vi "Single_Measurement_Main_v1.vi"(7 "Config files paths":T1={"ZI config file (.ini)"="Config_Ver_1\\Zurich_params.ini", "Keithley config file (.ini)"="Config_Ver_1\\Keithley_params.ini", "Arduino config file (.ini)"="Config_Ver_1\\pulse_sequence.ini"}, 8 "error in":errorcluster, 10 "Timeout [ms]":u64=5000, 11 "Resources In":T2 {"ZI ModHandle"."ModHandle" format="0x%08x"; "ZI ModHandle"."Conn" format="0x%08x"; "ZI Handle"."Handle" format="0x%08x"; "ZI Handle"."Conn" format="0x%08x"}) -> (0 "error out":errorcluster, 3 "Resources Out":T2 {"ZI ModHandle"."ModHandle" format="0x%08x"; "ZI ModHandle"."Conn" format="0x%08x"; "ZI Handle"."Handle" format="0x%08x"; "ZI Handle"."Conn" format="0x%08x"})   [LabVIEW 2021]
uses:
  Resources.ctl
  <instrlib>/Zurich Instruments LabOne/Public/ziTypeHandle.ctl
  <instrlib>/Zurich Instruments LabOne/Public/Modules/ziTypeModHandle.ctl
  Config_File_Paths.ctl
  <instrlib>/Keithley 622x LV 2009/Typedefs/KE622x -- On Off Control.ctl
  <vilib>/Utility/error.llb/Error Cluster From Error Code.vi
  <vilib>/ErrorRing/Error Ring.xnode
  <instrlib>/Zurich Instruments LabOne/Zurich Instruments LabOne.lvlib
  <instrlib>/Keithley 622x LV 2009/Keithley 622x.lvlib
panel:
  out "progress":dbl(slide) scale=0.0..1.0
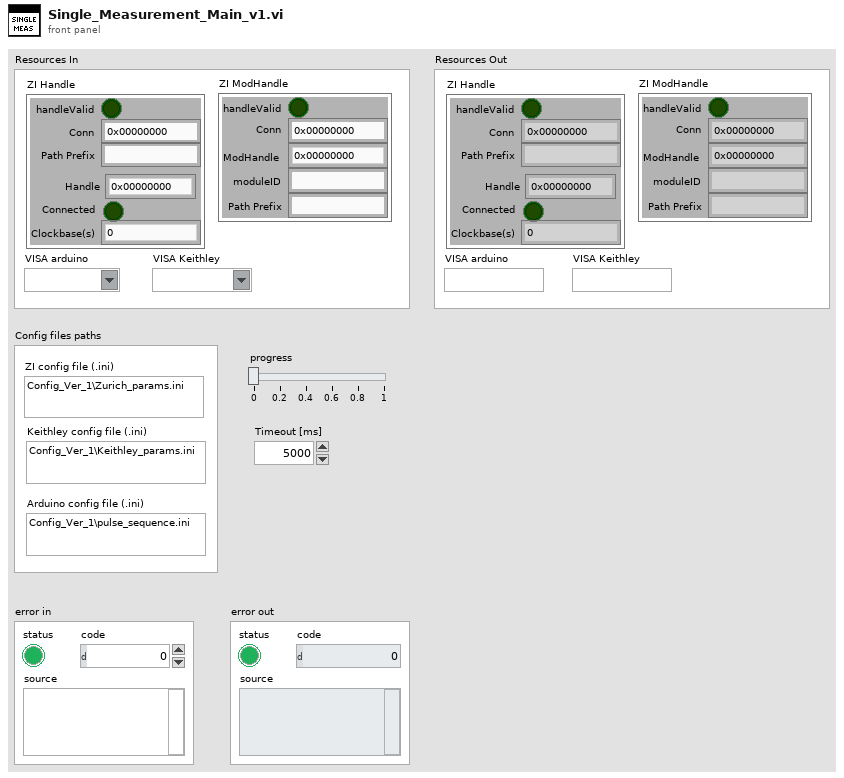
[diagram p1: front panel]
types:
  T1 = typedef "Config_File_Paths.ctl" = cluster{"ZI config file (.ini)":string, "Keithley config file (.ini)":string, "Arduino config file (.ini)":string}
  T2 = typedef "Resources.ctl" = cluster{"ZI Handle":T3, "ZI ModHandle":T4, "VISA arduino":refnum<visa-resource-name>, "VISA Keithley":refnum<visa-resource-name>}
  T3 = typedef "Zurich Instruments LabOne.lvlib/ziTypeHandle.ctl" = cluster{"handleValid":bool, "Conn":u64, "Path Prefix":string, "Handle":u64, "Connected":bool, "Clockbase(s)":dbl}
  T4 = typedef "Zurich Instruments LabOne.lvlib/ziTypeModHandle.ctl" = cluster{"handleValid":bool, "Conn":u64, "ModHandle":u64, "moduleID":string, "Path Prefix":string}
  T5 = typedef "Keithley 622x.lvlib/KE622x -- On Off Control.ctl" = enum16{"Off", "On"}
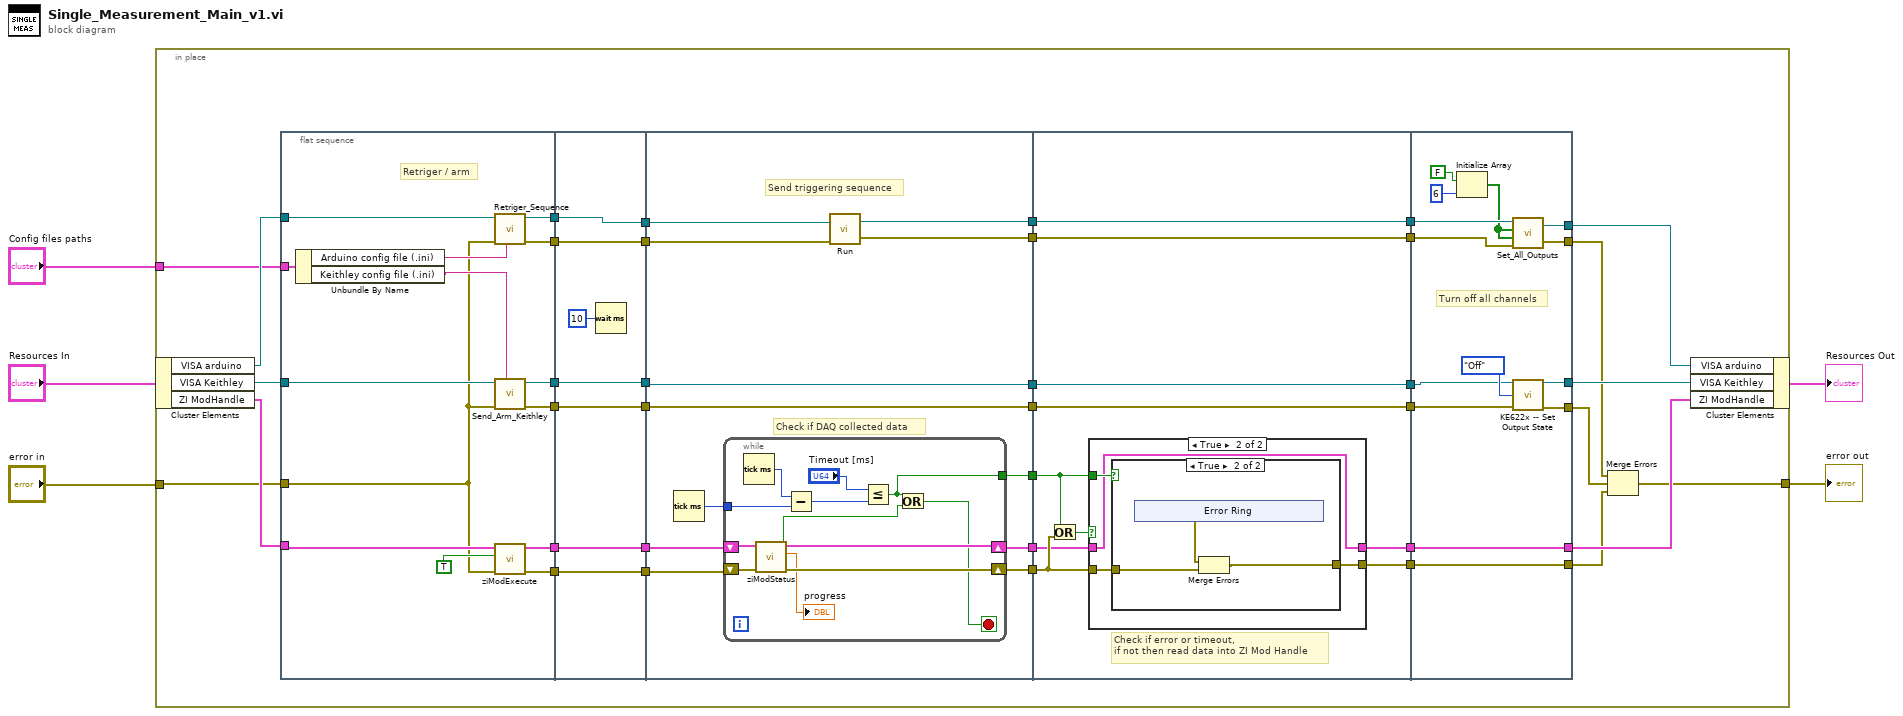
[diagram p0: block diagram]
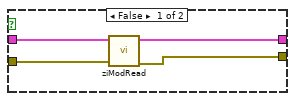
[diagram p2: hidden frame]
diagram:
  n1 = in-place {
    in-place-border: "Config files paths" -> [w39]
    in-place-border: "error in" -> [w38]
    in-place-border: [w6] -> w2
    n2 = in-place-cluster #1("Resources In") -> ("VISA arduino"=w40:refnum<visa-resource-name>, "VISA Keithley"=w41:refnum<visa-resource-name>, "ZI ModHandle"=w42:T4)
    n3 = flat-sequence {
      tunnel: w42 -> [w54]
      tunnel: w41 -> [w55]
      tunnel: w40 -> [w56]
      tunnel: w39 -> [w52]
      tunnel: w38 -> [w49]
      tunnel: [w48] -> w36
      tunnel: [w47] -> w34
      tunnel: [w46] -> w32
      tunnel: [w45] -> w30
      tunnel: [w44] -> w28
      tunnel: [w43] -> w26
      tunnel: [w62] -> w37
      tunnel: w36 -> [w62]
      tunnel: [w61] -> w35
      tunnel: w34 -> [w61]
      tunnel: [w60] -> w33
      tunnel: w32 -> [w60]
      tunnel: [w59] -> w31
      tunnel: w30 -> [w59]
      tunnel: [w58] -> w29
      tunnel: w28 -> [w58]
      tunnel: [w57] -> w27
      tunnel: w26 -> [w57]
      tunnel: w37 -> [w75]
      tunnel: w35 -> [w74]
      tunnel: w33 -> [w68]
      tunnel: w31 -> [w67]
      tunnel: w29 -> [w73]
      tunnel: w27 -> [w72]
      tunnel: [w70] -> w25
      tunnel: [w69] -> w24
      tunnel: [w68] -> w23
      tunnel: [w67] -> w22
      tunnel: [w66] -> w21
      tunnel: [w65] -> w20
      tunnel: [w64] -> w19
      tunnel: w25 -> [w97]
      tunnel: w24 -> [w96]
      tunnel: w23 -> [w95]
      tunnel: w22 -> [w94]
      tunnel: w21 -> [w91]
      tunnel: w20 -> [w90]
      tunnel: w19 -> [w92]
      tunnel: [w97] -> w18
      tunnel: [w96] -> w17
      tunnel: [w95] -> w16
      tunnel: [w94] -> w15
      tunnel: [w89] -> w14
      tunnel: [w88] -> w13
      tunnel: [w127] -> w9
      tunnel: [w128] -> w10
      tunnel: w18 -> [w121]
      tunnel: w17 -> [w119]
      tunnel: w16 -> [w125]
      tunnel: w15 -> [w124]
      tunnel: w14 -> [w128]
      tunnel: w13 -> [w127]
      tunnel: [w118] -> w11
      tunnel: [w117] -> w12
      tunnel: [w116] -> w7
      tunnel: [w115] -> w8
      frame #0 {
        # "Retriger / arm"
        n4 = Unbundle By Name(w52) -> ("Arduino config file (.ini)"=w51:string, "Keithley config file (.ini)"=w50:string)
        n5 = call "Retriger_Sequence.vi"("Filename (.ini)"=w51, "error in"=w49, "VISA arduino in"=w56) -> ("error out"=w48:errorcluster, "VISA arduino out"=w47:refnum<visa-resource-name>)  [unwired: 4 in, 3 out]
        n6 = call "Send_Arm_Keithley.vi"("Filename (.ini)"=w50, "error in"=w49, "Keithley VISA in"=w55) -> ("error out"=w45:errorcluster, "Keithley VISA out"=w46:refnum<visa-resource-name>)  [unwired: 6 in, 1 out]
        n7 = call <instrlib>:"ziModExecute.vi"("Error In"=w49, "Modal (F)"=TRUE, "ziModHandle In"=w54) -> ("Error Out"=w43:errorcluster, "ziModHandle Out"=w44:T4)  [unwired: 6 in]
      }
      frame #1 {
        n8 = Wait (ms)(milliseconds to wait=u32 10) -> ()  [unwired: 1 out]
      }
      frame #2 {
        # "Check if DAQ collected data"
        # "Send triggering sequence"
        n9 = Tick Count (ms)() -> (millisecond timer value=w71:u32)
        n10 = while {
          shift-right: [w86] -> w65
          shift-left: w73 -> [w87]
          shift-right: [w84] -> w64
          shift-left: w72 -> [w85]
          tunnel: w71 -> [w81]
          tunnel: [w76] -> w66
          stop <- w77 stop-if-true
          n11 = Tick Count (ms)() -> (millisecond timer value=w82:u32)
          n12 = call <instrlib>:"ziModStatus.vi"("Error In"=w85, "ModHandle IN"=w87) -> ("Error Out"=w84:errorcluster, "Finished?"=w78:bool, "Progress (unity)"=→"progress":dbl, "ModHandle Out"=w86:T4)  [unwired: 5 in]
          n13 = Subtract(x=w82, y=w81) -> (x-y=w80:u32)
          n14 = Less Or Equal?(x="Timeout [ms]", y=w80) -> (x <= y?=w76:bool)
          n15 = Or(x=w76, y=w78) -> (x .or. y?=w77:bool)
        }
        n16 = call "Run.vi"("error in"=w75, "VISA arduino in"=w74) -> ("error out"=w69:errorcluster, "VISA arduino out"=w70:refnum<visa-resource-name>)  [unwired: 1 in]
      }
      frame #3 {
        # "Check if error or timeout,\nif not then read data into ZI Mod Handle"
        n17 = Or(x=w91, y=w92) -> (x .or. y?=w93:bool)
        n18 = case shown="True" w93 {
          tunnel: w92 -> [w100 w104]
          tunnel: w91 -> [_ w105]
          tunnel: [w99 w103] -> w88
          tunnel: w90 -> [w101 w102]
          tunnel: [w98 w102] -> w89
          frame False {
            n19 = call <instrlib>:"ziModRead.vi"("error in"=w100, "ziModHandle In"=w101) -> ("error out"=w99:errorcluster, "ziModHandle Out"=w98:T4)  [unwired: 8 in]
          }
          frame True {
            n20 = case shown="True" w105 {
              tunnel: w104 -> [w106 w108]
              tunnel: [w106 w107] -> w103
              frame False {
              }
              frame True {
                n21 = xnode "Error Ring"() -> ("error out"=w109:errorcluster)
                n22 = Merge Errors(w109, w108) -> (w107:errorcluster)
              }
            }
          }
        }
      }
      frame #4 {
        # "Turn off all channels"
        n23 = Initialize Array(FALSE, 6 ("dimension size")) -> (w120:bool[])
        n24 = call "Set_All_Outputs.vi"("error in"=w119, "register 2 (8-13)"=w120, "register 1 (2-7)"=w120, "VISA arduino in"=w121) -> ("error out"=w116:errorcluster, "VISA arduino out"=w117:refnum<visa-resource-name>)
        n25 = call <instrlib>:"KE622x -- Set Output State.vi"("Resource In"=w125, "Output State"=KE622x_--_On_Off_Control."Off", "error in (no error)"=w124) -> ("Resource Out (dupl)"=w118:refnum<visa-resource-name>, "error out"=w115:errorcluster)  [unwired: 11 in]
      }
    }
    n26 = Merge Errors(w7, w8, w9) -> (w6:errorcluster)
    n27 = in-place-cluster #1("VISA arduino"=w12, "VISA Keithley"=w11, "ZI ModHandle"=w10) -> (→"Resources Out":T2)
  }
  "error out" <- w2
